vi "VIBRATION SENSOR INTERLOCK.vi"(1 "Operating Vibration Value":dbl, 2 "Critical Vibration Value":dbl) -> (0 "Alarm":bool)   [LabVIEW 2014]
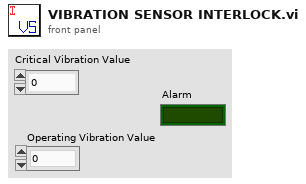
[diagram p1: front panel]
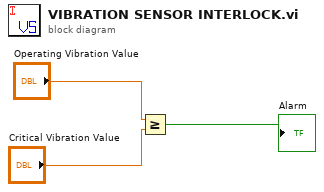
[diagram p0: block diagram]
diagram:
  n1 = Greater Or Equal?(x="Operating Vibration Value", y="Critical Vibration Value") -> (x >= y?=→"Alarm":bool)
